vi "UserInput.vi"() -> (2 "Points per Iteration":dbl format="%#g", 3 "Number of Iterations":dbl format="%#g")   [LabVIEW 2014]
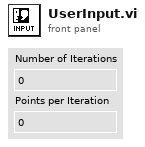
[diagram p1: front panel]
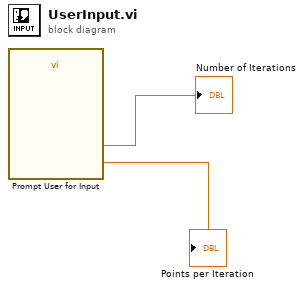
[diagram p0: block diagram]
diagram:
  n1 = call "Prompt User for Input"() -> ("Points per Iteration"=→"Points per Iteration":dbl, "Number of Iterations"=→"Number of Iterations":dbl)  [unwired: 16 in, 2 out]
